vi "Build Pulse Train.vi"(7 "method":i32(ring)=1 items=["nearest", "linear", "spline", "cubic Hermite"], 8 "prototype spec":T1={"Prototype Pulse"=[], "delta t of Prototype Pulse"=0.1}, 9 "Delay":dbl[](array[numeric]), 10 "Amplitude":dbl[](array[numeric]), 11 "X":dbl[](array[numeric])) -> (0 "error":i32, 3 "Pulse Train":dbl[](array[numeric]))   [LabVIEW 2020, in "NI_AALBase.lvlib"]
uses:
  NI_AALBase.lvlib
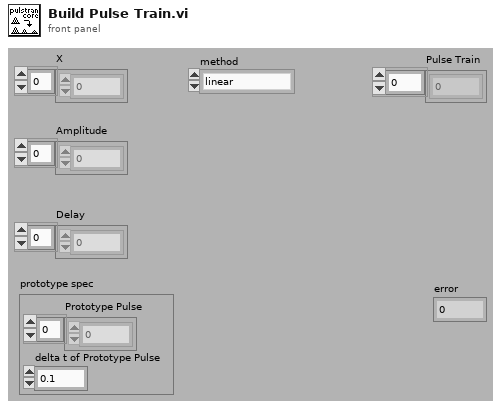
[diagram p1: front panel]
types:
  T1 = cluster{"Prototype Pulse":dbl[], "delta t of Prototype Pulse":dbl}
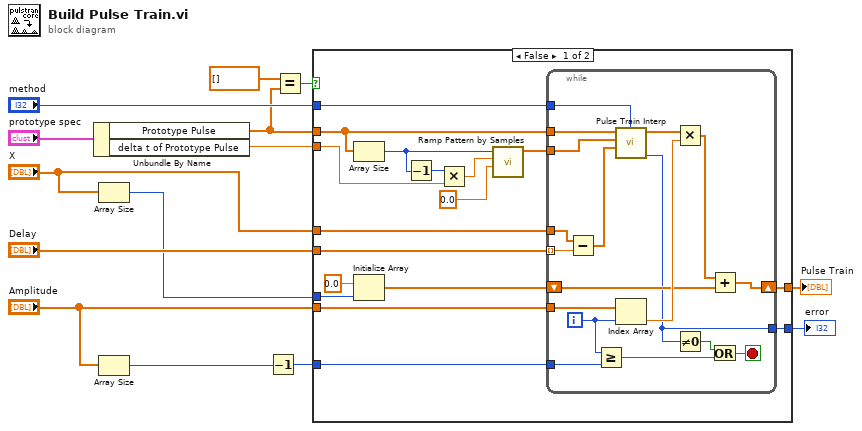
[diagram p0: block diagram]
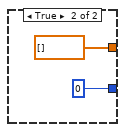
[diagram p2: hidden frame]
diagram:
  n1 = Unbundle By Name("prototype spec") -> ("Prototype Pulse"=w2:dbl[], "delta t of Prototype Pulse"=w6:dbl)
  n2 = Array Size(array="X") -> (size(s)=w5:i32)
  n3 = Array Size(array="Amplitude") -> (size(s)=w9:i32)
  n4 = Decrement(x=w9) -> (x-1=w4:i32)
  n5 = Equal?(x=dbl[] [], y=w2) -> (x = y?=w3:bool)
  n6 = case shown="False" w3 {
    tunnel: [w31 dbl[] []] -> w14
    tunnel: "Delay" -> [w30 _]
    tunnel: [w29 0] -> w12
    tunnel: "method" -> [w28 _]
    tunnel: w4 -> [w27 _]
    tunnel: "X" -> [w26 _]
    tunnel: "Amplitude" -> [w25 _]
    tunnel: w2 -> [w24 _]
    tunnel: w6 -> [w20 _]
    tunnel: w5 -> [w16 _]
    frame False {
      n7 = Array Size(array=w24) -> (size(s)=w21:i32)
      n8 = Initialize Array(0.0, w16) -> (w15:dbl[])
      n9 = Decrement(x=w21) -> (x-1=w22:i32)
      n10 = Multiply(x=w22, y=w20) -> (x*y=w23:dbl)
      n11 = call "Ramp Pattern by Samples.vi"("start"=0.0, "end"=w23, "samples"=w21) -> ("Ramp Pattern"=w18:dbl[])  [unwired: 7 in, 1 out]
      n12 = while {
        tunnel: w30 -> [w34] mode=indexing
        tunnel: w24 -> [w46]
        tunnel: w26 -> [w33]
        shift-right: [w49] -> w31
        shift-left: w15 -> [w37]
        tunnel: w25 -> [w48]
        tunnel: w27 -> [w39]
        tunnel: w18 -> [w45]
        tunnel: [w36] -> w29
        tunnel: w28 -> [w35]
        i -> [w40]
        stop <- w47 stop-if-true
        n13 = Subtract(x=w33, y=w34) -> (x-y=w32:dbl[])
        n14 = Greater Or Equal?(x=w40, y=w39) -> (x >= y?=w44:bool)
        n15 = call "Pulse Train Interp.vi"("method"=w35, "Xi"=w32, "X"=w45, "Y"=w46) -> ("error"=w36:i32, "Yi"=w42:dbl[])  [unwired: 5 in, 1 out]
        n16 = Index Array(array=w48, index=w40) -> (element=w41:dbl)
        n17 = Multiply(x=w42, y=w41) -> (x*y=w38:dbl[])
        n18 = Not Equal To 0?(x=w36) -> (x != 0?=w43:bool)
        n19 = Add(x=w38, y=w37) -> (x+y=w49:dbl[])
        n20 = Or(x=w43, y=w44) -> (x .or. y?=w47:bool)
      }
    }
    frame True {
    }
  }
  "Pulse Train" <- w14
  "error" <- w12
